vi "Unload.vi"(8 "error in":errorcluster, 11 "CameraTool in":refnum<class "CameraTool Class.lvclass">) -> (0 "error out":errorcluster, 3 "Gantry out":refnum<class "Gantry Class.lvclass">)   [LabVIEW 2011, in "CameraTool Class.lvclass"]
uses:
  CameraTool Class.lvclass
  Gantry Class/Gantry Class.lvclass
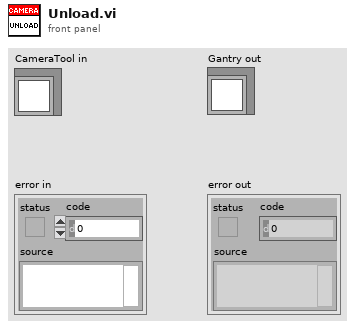
[diagram p1: front panel]
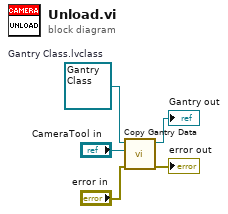
[diagram p0: block diagram]
diagram:
  w3 = refnum<class "Gantry Class.lvclass"> refnum  # Gantry Class.lvclass
  n1 = call "Copy Gantry Data.vi"("error in"="error in", "Gantry Source"="CameraTool in", "Gantry Dest"=w3) -> ("error out"=→"error out":errorcluster, "Gantry Result"=→"Gantry out":refnum<class "Gantry Class.lvclass">)  [unwired: 7 in]
